vi "Post action.vi"(1 "PostAction":T1=enum."Do Nothing", 2 "Scan Parameters":T2={"DAQ Channel"=3, "Label"="\nappliedVsg2=", "Start"=-0.01, "End"=0.4, "Step"=0.01, "rate"=0.01} {"rate" format="%.2f"; "Step" format="%#_6p"; "End" format="%#_6p"; "Start" format="%#_6p"}, 3 "Index":i32=41) -> ()   [LabVIEW 2016]
uses:
  Typedefs/Cluster - ScanParamters.ctl
  Typedefs/Enum - PostAction.ctl
  <userlib>/LevyLab/DAQ-Lockin-SubVI/Lockin-4461_MultiChannel - IV 3.0 globals.vi
panel:
  in  "milliseconds to wait":u32=10000
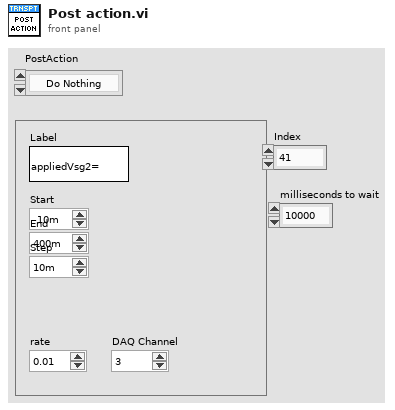
[diagram p1: front panel]
types:
  T1 = typedef "Enum - PostAction.ctl" = enum16{"Clear DAQ Tasks", "Check Temperature", "Wait", "Do Nothing"}
  T2 = typedef "Cluster - ScanParamters.ctl" = cluster{"DAQ Channel":i32, "Label":string, "Start":dbl, "End":dbl, "Step":dbl, "rate":dbl}
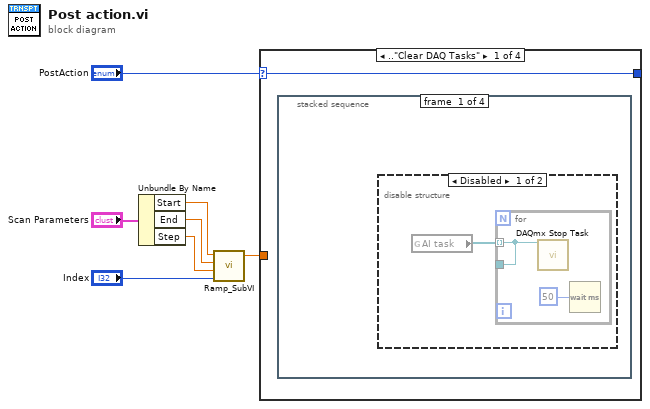
[diagram p0: block diagram]
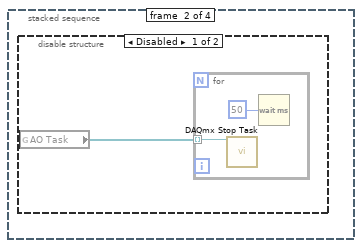
[diagram p3: hidden frame]
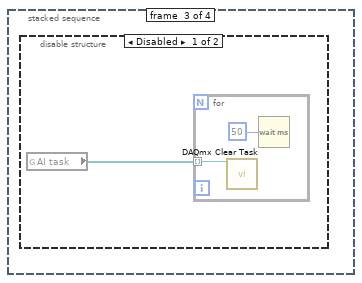
[diagram p5: hidden frame]
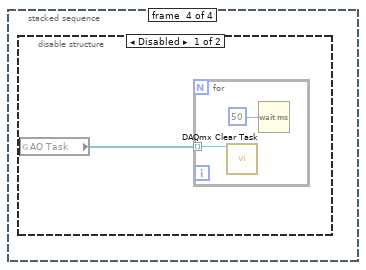
[diagram p7: hidden frame]
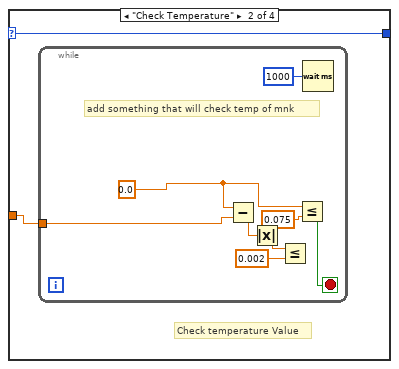
[diagram p9: hidden frame]
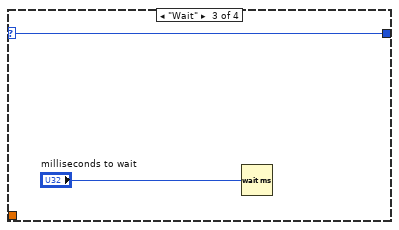
[diagram p10: hidden frame]
diagram:
  n1 = Unbundle By Name("Scan Parameters") -> ("Start"=w3:dbl, "End"=w2:dbl, "Step"=w1:dbl)
  n2 = call <userlib>:"Ramp_SubVI.vi"("index"="Index", "step"=w1, "end"=w2, "start"=w3) -> ("Numeric"=w6:dbl)  [unwired: 1 in, 1 out]
  n3 = case shown="..\"Clear DAQ Tasks\"" "PostAction" {
    tunnel: w6 -> [_ w22 _ _]
    selector: "PostAction" -> [w8 w21 w32 w33]
    tunnel: [w8 w21 w32 w33] -> _
    frame .."Clear DAQ Tasks" {
      n4 = stacked-sequence {
        frame #0 {
          n5 = disable-structure shown="Disabled" {
            frame Disabled {
              n6 = global read "Lockin-4461_MultiChannel - IV 3.0 globals.vi" "AI task"() -> (w9:refnum<k21>[])
              n7 = for {
                tunnel: w9 -> [w10] mode=indexing
                tunnel: [w10] -> _
                n8 = call <vilib>:"DAQmx Stop Task.vi"("task/channels in"=w10) -> ()  [unwired: 13 in, 2 out]
                n9 = Wait (ms)(milliseconds to wait=u32 50) -> ()  [unwired: 1 out]
              }
            }
            frame Enabled {
            }
          }
        }
        frame #1 {
          n10 = disable-structure shown="Disabled" {
            frame Disabled {
              n11 = global read "Lockin-4461_MultiChannel - IV 3.0 globals.vi" "AO Task"() -> (w12:refnum<k21>[])
              n12 = for {
                tunnel: w12 -> [w14] mode=indexing
                n13 = call <vilib>:"DAQmx Stop Task.vi"("task/channels in"=w14) -> ()  [unwired: 13 in, 2 out]
                n14 = Wait (ms)(milliseconds to wait=u32 50) -> ()  [unwired: 1 out]
              }
            }
            frame Enabled {
            }
          }
        }
        frame #2 {
          n15 = disable-structure shown="Disabled" {
            frame Disabled {
              n16 = global read "Lockin-4461_MultiChannel - IV 3.0 globals.vi" "AI task"() -> (w15:refnum<k21>[])
              n17 = for {
                tunnel: w15 -> [w17] mode=indexing
                n18 = call <vilib>:"DAQmx Clear Task.vi"("task in"=w17) -> ()  [unwired: 14 in, 1 out]
                n19 = Wait (ms)(milliseconds to wait=u32 50) -> ()  [unwired: 1 out]
              }
            }
            frame Enabled {
            }
          }
        }
        frame #3 {
          n20 = disable-structure shown="Disabled" {
            frame Disabled {
              n21 = global read "Lockin-4461_MultiChannel - IV 3.0 globals.vi" "AO Task"() -> (w18:refnum<k21>[])
              n22 = for {
                tunnel: w18 -> [w20] mode=indexing
                n23 = call <vilib>:"DAQmx Clear Task.vi"("task in"=w20) -> ()  [unwired: 14 in, 1 out]
                n24 = Wait (ms)(milliseconds to wait=u32 50) -> ()  [unwired: 1 out]
              }
            }
            frame Enabled {
            }
          }
        }
      }
    }
    frame "Check Temperature" {
      # "Check temperature Value"
      n25 = while {
        tunnel: w22 -> [w26]
        stop <- w24 stop-if-true
        w23 = 0.0 ("y")
        # "add something that will check temp of mnk"
        n26 = Subtract(x=w23, y=w26) -> (x-y=w30:dbl)
        n27 = Absolute Value(x=w30) -> (abs(x)=w29:dbl)
        n28 = Less Or Equal?(x=w29, y=0.002) -> ()  [unwired: 1 out]
        n29 = Less Or Equal?(x=w23, y=0.075) -> (x <= y?=w24:bool)
        n30 = Wait (ms)(milliseconds to wait=u32 1000) -> ()  [unwired: 1 out]
      }
    }
    frame "Wait" {
      n31 = Wait (ms)(milliseconds to wait="milliseconds to wait") -> ()  [unwired: 1 out]
    }
    frame "Do Nothing".. {
      # "Do nothing"
    }
  }
